vi "Teleop.vi"(10 "Match Info":T1={"Autonomous Elapsed Seconds"=0.0, "TeleOp Elapsed Seconds"=0.0, "Disabled Elapsed Seconds"=0.0, "Visited Autonomous"=FALSE, "Visited TeleOp"=FALSE, "Visited Disabled"=FALSE, "Autonomous Settings"={"Autonomous Style"=enum."Independent", "VI Refnum"=refnum}}, 11 "Call Context":T2) -> ()   [LabVIEW 2014]
doc: "This VI is called for each TeleOp packet received from the DS where the robot is not disabled. It is often used to read from the joysticks and update I/O or to update setpoints for timed control loops. It should complete and return within 20 milliseconds or it may miss DS packets."
uses:
  <vilib>/Rock Robotics/WPI/DriverStation/WPI_DriverStationDerivedRobotMode.ctl
  <vilib>/Rock Robotics/WPI/DriverStation/WPI_DriverStationMatch Info.ctl
  Lift Command.ctl
  Drivetrain Command.ctl
  Intake Command.ctl
  <vilib>/Rock Robotics/WPI/Joystick/WPI_JoystickGetSetRefNum.vi
  <vilib>/Rock Robotics/Network Tables/SD Read Boolean.vi
  <vilib>/Rock Robotics/Network Tables/SD Read Number.vi
  Robot Global Data.vi
panel:
  out "Sample Slider 0":dbl(slide) scale=0.0..5.0
  out "Sample Boolean 1":bool
  out "Sample Boolean 0":bool
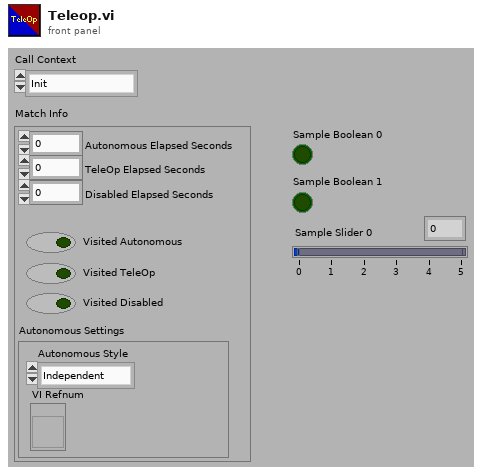
[diagram p1: front panel]
types:
  T1 = typedef "WPI_DriverStationMatch Info.ctl" = cluster{"Autonomous Elapsed Seconds":dbl, "TeleOp Elapsed Seconds":dbl, "Disabled Elapsed Seconds":dbl, "Visited Autonomous":bool, "Visited TeleOp":bool, "Visited Disabled":bool, "Autonomous Settings":cluster{"Autonomous Style":enum16{"Iterative", "Independent"}, "VI Refnum":refnum<vi>}}
  T2 = typedef "WPI_DriverStationDerivedRobotMode.ctl" = enum16{"Init", "Execute", "Stop"}
  T3 = typedef "Intake Command.ctl" = cluster{"Closed":bool, "Left Speed":dbl, "Right Speed":dbl}
  T4 = typedef "Drivetrain Command.ctl" = cluster{"X":dbl, "\nY":dbl}
  T5 = typedef "Lift Command.ctl" = cluster{"Lift Speed":dbl}
  T6 = typedef "WPI_JoystickDevRef.ctl" = cluster{"Device":T7}
  T7 = typedef "WPI_JoystickDeviceEnum.ctl" = enum16{"USB 0", "USB 1", "USB 2", "USB 3", "USB 4", "USB 5"}
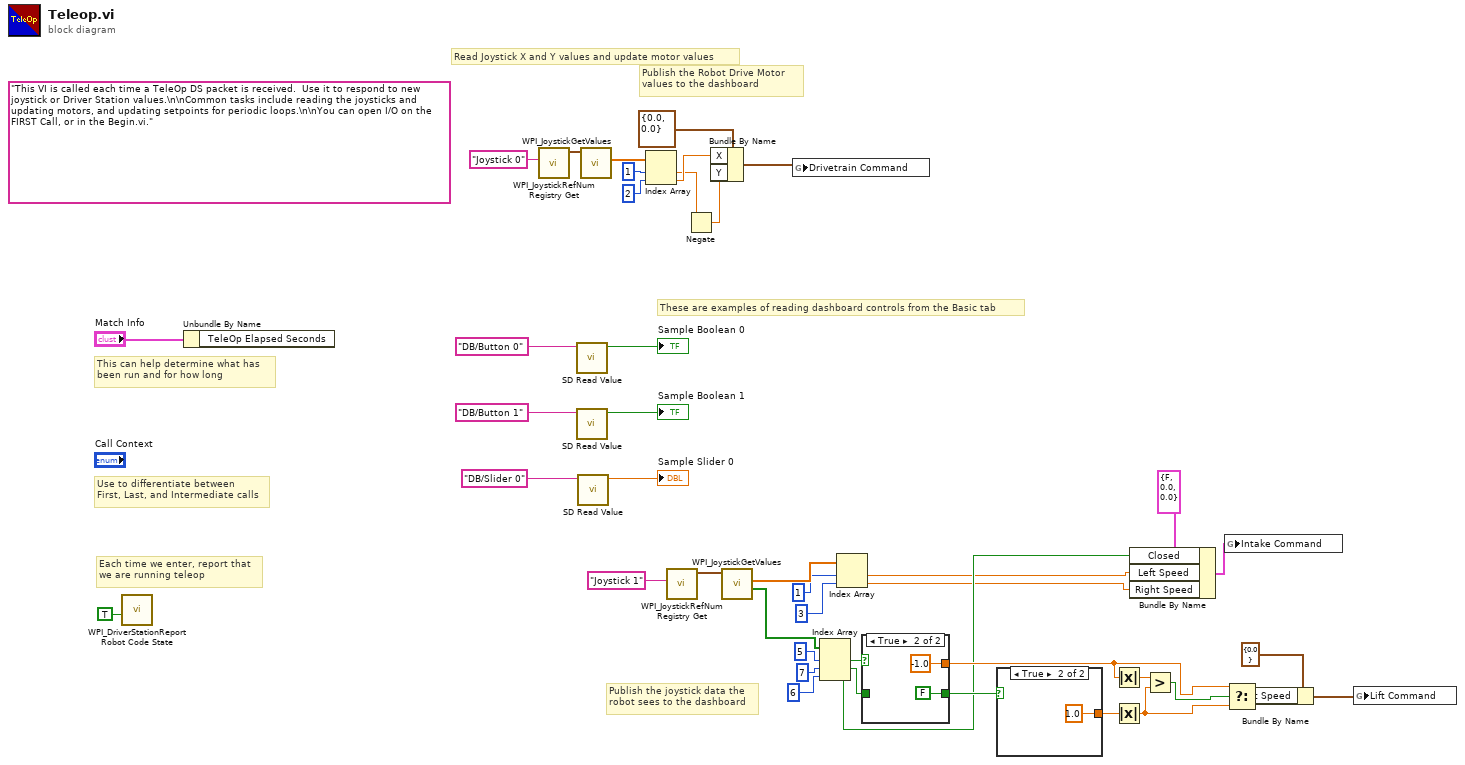
[diagram p0: block diagram]
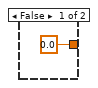
[diagram p2: hidden frame]
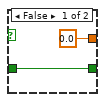
[diagram p3: hidden frame]
diagram:
  (unwired) "This VI is called each time a TeleOp DS packet is received.  Use it to respond to new joystick or Driver Station values.\n\nCommon tasks include reading the joysticks and updating motors, and updating setpoints for periodic loops.\n\nYou can open I/O on the FIRST Call, or in the Begin.vi."
  # "These are examples of reading dashboard controls from the Basic tab"
  # "Publish the Robot Drive Motor\nvalues to the dashboard"
  # "Publish the joystick data the\nrobot sees to the dashboard"
  # "Each time we enter, report that\nwe are running teleop"
  # "Use to differentiate between\nFirst, Last, and Intermediate calls"
  # "This can help determine what has\nbeen run and for how long"
  # "Read Joystick X and Y values and update motor values"
  n1 = call <vilib>:"WPI_DriverStationReport Robot Code State.vi"("TeleOp"=TRUE ("Autonomous")) -> ()  [unwired: 10 in, 1 out]
  n2 = Unbundle By Name("Match Info") -> ()  [unwired: 1 out]
  n3 = call <vilib>:"WPI_JoystickRefNum Registry Get.vi"("refnum name"="Joystick 0") -> ("JoystickDevRef"=w41:T6)  [unwired: 1 in, 9 out]
  n4 = call-poly <vilib>:"SD Read Value.vi"("Name"="DB/Button 0" ("refnum name")) -> ("Boolean"=→"Sample Boolean 0":bool)  [unwired: 8 in, 2 out]
  n5 = call-poly <vilib>:"SD Read Value.vi"("Name"="DB/Button 1" ("refnum name")) -> ("Boolean"=→"Sample Boolean 1":bool)  [unwired: 8 in, 2 out]
  n6 = call-poly <vilib>:"SD Read Value.vi"("Name"="DB/Slider 0" ("refnum name")) -> ("Numeric"=→"Sample Slider 0":dbl)  [unwired: 8 in, 2 out]
  n7 = call <vilib>:"WPI_JoystickGetValues.vi"("JoystickDevRef"=w41) -> ("Axes"=w33:dbl[])  [unwired: 6 in, 4 out]
  n8 = Index Array(array=w33, index #1=1 ("index"), index #2=2 ("index")) -> (element #1=w2:dbl, element #2=w16:dbl)
  n9 = call <vilib>:"WPI_JoystickRefNum Registry Get.vi"("refnum name"="Joystick 1") -> ("JoystickDevRef"=w31:T6)  [unwired: 1 in, 9 out]
  n10 = Negate(x=w2) -> (-x=w1:dbl)
  n11 = Bundle By Name(cluster=T4 {"X"=0.0, "\nY"=0.0} ("Drivetrain Command"), "X"=w16, "Y"=w1) -> (w14:T4)
  n12 = call <vilib>:"WPI_JoystickGetValues.vi"("JoystickDevRef"=w31) -> ("Buttons"=w30:bool[], "Axes"=w7:dbl[])  [unwired: 6 in, 3 out]
  n13 = global write "Robot Global Data.vi" "Drivetrain Command"(w14) -> ()
  n14 = Index Array(array=w30, index #1=5 ("index"), index #2=7 ("index"), index #3=6 ("index")) -> (element #1=w27:bool, element #2=w25:bool, element #3=w8:bool)
  n15 = Index Array(array=w7, index #1=1 ("index"), index #2=3 ("index")) -> (element #1=w4:dbl, element #2=w3:dbl)
  n16 = case shown="True" w27 {
    tunnel: [w45 FALSE] -> w26
    tunnel: w25 -> [w45 _]
    tunnel: [0.0 -1.0] -> w22
    frame False {
    }
    frame True {
    }
  }
  n17 = case shown="True" w26 {
    tunnel: [0.0 1.0] -> w24
    frame False {
    }
    frame True {
    }
  }
  n18 = Absolute Value(x=w22) -> (abs(x)=w23:dbl)
  n19 = Absolute Value(x=w24) -> (abs(x)=w21:dbl)
  n20 = Bundle By Name(cluster=T3 {"Closed"=FALSE, "Left Speed"=0.0, "Right Speed"=0.0} ("Intake Command"), "Closed"=w8, "Left Speed"=w4, "Right Speed"=w3) -> (w9:T3)
  n21 = Greater?(x=w23, y=w21) -> (0:w20:bool)
  n22 = global write "Robot Global Data.vi" "Intake Command"(w9) -> ()
  n23 = Select(t=w22, s=w20, f=w21) -> (s? t:f=w19:dbl)
  n24 = Bundle By Name(cluster=T5 {"Lift Speed"=0.0} ("Lift Command"), "Lift Speed"=w19) -> (w17:T5)
  n25 = global write "Robot Global Data.vi" "Lift Command"(w17) -> ()
